vi "PH_ImageOperator.PC Set FF Settings.vi"(0 "i ref in":refnum<vi>, 1 "Calc Fill Factor":bool, 2 "Filter":bool, 3 "Threshold":dbl, 4 "Damage Threshold [J/cm²]":dbl, 5 "error in (no error)":errorcluster) -> (14 "i ref out":refnum<vi>, 19 "error out":errorcluster)   [LabVIEW 2014, in "PH_ImageOperator.lvlib"]
doc: "This VI writes the Fill Factor Measurement settings to own attributes and sets the GUI elements."
uses:
  PH_ImageOperator.lvlib
  PH_Common/PH_Common.lvlib
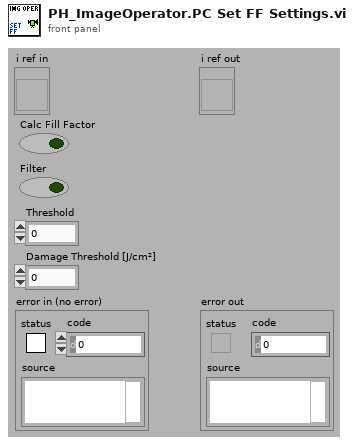
[diagram p1: front panel]
types:
  T1 = typedef "PH_ImageOperator.lvlib/PH_ImageOperator.i attribute.ctl" = cluster{"GUI Refs":cluster{"Delete":refnum<vi>, "Calibration status":refnum<vi>, "BI subtracted":refnum<vi>, "calc Energy":refnum<vi>, "Energy: expected value":refnum<vi>, "Energy: Tolerance":refnum<vi>, "Energy calculated":refnum<vi>, "Energy":refnum<vi>, "calc Beam Anal":refnum<vi>, "Maj Diam 1/esquare":refnum<vi>, "Min Diam 1/esquare":refnum<vi>, "Azi Angle":refnum<vi>, "Min/Maj Diam esquare":refnum<vi>, "Beam analysed":refnum<vi>, "CoG - x":refnum<vi>, "CoG - y":refnum<vi>, "BA: Method":refnum<vi>, "BA: Steps":refnum<vi>, "BA: Factor":refnum<vi>, "calc Traces":refnum<vi>, "Traces: Fit Gauss":refnum<vi>, "Traces calculated":refnum<vi>, "Maj FWHM":refnum<vi>, "Min FWHM":refnum<vi>, "Major Trace":refnum<vi>, "Minor Trace":refnum<vi>, "Maj Fit Order":refnum<vi>, "Min Fit Order":refnum<vi>, "Position calculated":refnum<vi>, "Position":refnum<vi>, "Type":refnum<vi>, "Center":refnum<vi>, "exp - X":refnum<vi>, "exp - Y":refnum<vi>, "Tolerance":refnum<vi>, "f":refnum<vi>, "M":refnum<vi>, "D":refnum<vi>, "q":refnum<vi>, "Dummy Method":refnum<vi>, "Dummy Type":refnum<vi>, "Global On":refnum<vi>, "Traces: No offset":refnum<vi>, "Maj 99%":refnum<vi>, "Min 99%":refnum<vi>, "GUI FF Image":refnum<vi>, "calc Fill Factor":refnum<vi>, "FF calculated":refnum<vi>, "Fill Factor: Filter?":refnum<vi>, "FF: Damage Threshold":refnum<vi>, "FF: Threshold":refnum<vi>, "FF: max allow. Energy":refnum<vi>, "FF: Fillfactor":refnum<vi>, "Calibration data":refnum<vi>}, "List of GUIs":string[], "Calibration":cluster{"Status":T2, "Calibration data":T3, "Calibration Data File":path}, "Final Image":cluster{"BI Subtraction Failure":bool}, "Energy":cluster{"on":bool, "expected value [mJ]":dbl, "Tolerance [%]":dbl, "State":T2, "Energy [mJ]":dbl, "Unit":string, "calculated @":timestamp}, "Beam Analysis":cluster{"on":bool, "Data":T4, "Method":bool, "Steps":i32, "Factor":i32, "ROI":cluster{"Left":i32, "Top":i32, "Right":i32, "Bottom":i32}, "analysed @":timestamp}, "Trace Analysis":cluster{"on":bool, "Fit on":bool, "Maj FWHM":dbl, "Min FWHM":dbl, "Maj Fit Order":i32, "Min Fit Order":i32, "No Offset":bool, "Maj 99%":dbl, "Min 99%":dbl, "Traces":cluster{"XScaleName":string, "Y Scale Minimum":sgl, "Y Scale Maximum":sgl, "X Scale Minimum":sgl, "X Scale Maximum":sgl, "Traces":cluster{"Index":sgl[], "Trace":dbl[]}[]}[], "analysed @":timestamp}, "Position Analysis":cluster{"on":bool, "exp - X":i32, "exp - Y":i32, "focal length [mm]":dbl, "Magnification":dbl, "Delta":dbl, "Theta":dbl, "Tolerance":dbl, "Type":bool, "analysed @":timestamp}, "Fill Factor":cluster{"on":bool, "Filter on?":bool, "Threshold":dbl, "Damage Threshold [J/cm²]":dbl, "Fillfactor":dbl, "Max. allowed Energy [J]":dbl, "calculated @":timestamp}, "Statistician Service ID":i32, "Images":cluster{"Background":T5, "OP":T5, "GUI":T5, "BA: ROI":T5, "Trace: Turn":T5, "FF: Main":T5, "FF: Help":T5, "PSDB: BG":T5, "PSDB: OP":T5, "PSDB: FF":T5}}
  T2 = typedef "PH_StatusHandler.lvlib/PH_StatusHandler.Status.ctl" = i16
  T3 = typedef "PH_ImageCalibrator.lvlib/PH_ImageCalibrator.Calibration Data.ctl" = cluster{"Date":string, "Time":string, "Cam Settings":cluster{"Cam ID":string, "Gain":dbl, "Brightness":dbl, "Shutter":dbl, "Cam Error":bool, "Mode":i32}, "Background Image":cluster{"Image":dbl[][], "Image Error":bool}, "Linear Calibration":cluster{"Calibration Factor":dbl, "not mm or mrad":bool}, "Energy Calibration":cluster{"Calibration Factor":dbl, "no mJ":bool}}
  T4 = typedef "PH_ImageOperator.lvlib/PH_ImageOperator.Beam Analysis Data.ctl" = cluster{"CoG-x":sgl, "CoG-y":sgl, "Maj Dim":dbl, "Min Dim":dbl, "Ellipticity":dbl, "Azimuth Angle [rad]":dbl, "Azi Angle rel to Maj?":bool}
  T5 = typedef "IMAQ Image.ctl" = refnum<image>
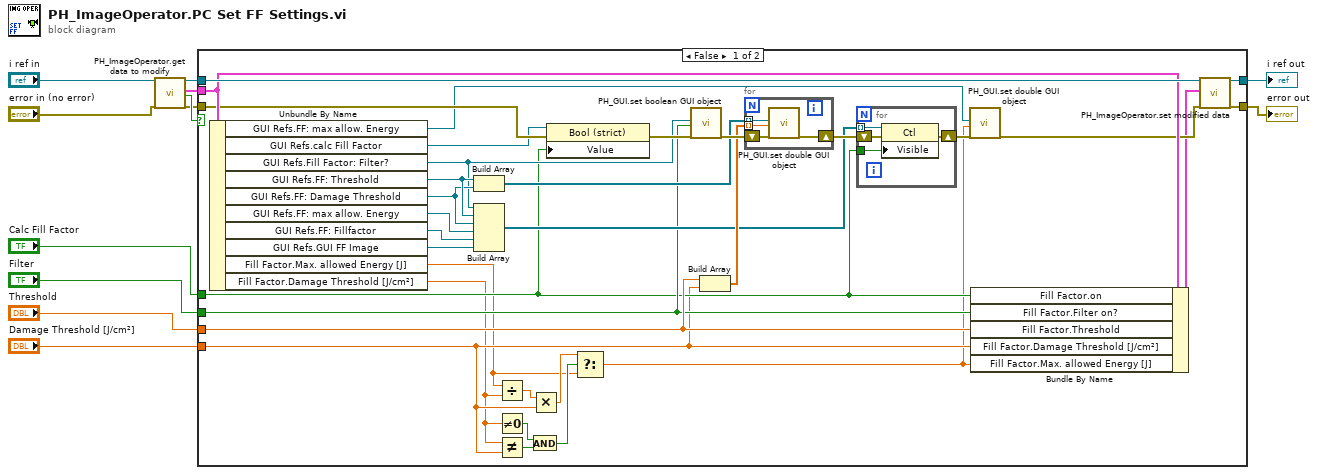
[diagram p0: block diagram]
diagram:
  n1 = call "PH_ImageOperator.get data to modify.vi"("i ref in"="i ref in", "error in (no error)"="error in (no error)") -> ("i ref out"=w4:refnum<vi>, "i attribute"=w9:T1, "timed out"=w8:bool, "error out"=w3:errorcluster)  [unwired: 14 in]
  n2 = case shown="False" w8 {
    tunnel: w3 -> [w32 w55]
    tunnel: w4 -> [w46 w56]
    tunnel: [w45 w56] -> w5
    tunnel: [w44 w55] -> w7
    tunnel: w9 -> [w43 _]
    tunnel: "Calc Fill Factor" -> [w27 _]
    tunnel: "Threshold" -> [w42 _]
    tunnel: "Damage Threshold [J/cm²]" -> [w24 _]
    tunnel: "Filter" -> [w29 _]
    frame False {
      n3 = Unbundle By Name(w43) -> ("GUI Refs.FF: max allow. Energy"=w18:refnum<vi>, "GUI Refs.calc Fill Factor"=w30:refnum<vi>, "GUI Refs.Fill Factor: Filter?"=w28:refnum<vi>, "GUI Refs.FF: Threshold"=w37:refnum<vi>, "GUI Refs.FF: Damage Threshold"=w36:refnum<vi>, "GUI Refs.FF: max allow. Energy"=w35:refnum<vi>, "GUI Refs.FF: Fillfactor"=w34:refnum<vi>, "GUI Refs.GUI FF Image"=w26:refnum<vi>, "Fill Factor.Max. allowed Energy [J]"=w13:dbl, "Fill Factor.Damage Threshold [J/cm²]"=w23:dbl)
      n4 = Build Array(w37, w36) -> (w39:refnum<vi>[])
      n5 = Build Array(w28, w37, w36, w35, w34, w26) -> (w33:refnum<vi>[])
      n6 = Divide(x=w13, y=w23) -> (x/y=w21:dbl)
      n7 = Not Equal To 0?(x=w23) -> (x != 0?=w22:bool)
      n8 = Not Equal?(x=w23, y=w24) -> (x != y?=w25:bool)
      n9 = And(x=w22, y=w25) -> (x .and. y?=w16:bool)
      n10 = Multiply(x=w21, y=w24) -> (x*y=w15:dbl)
      n11 = property class="Bool (strict)"(reference=w30, error in=w32, "Value"=w27) -> (error out=w31:errorcluster)  [unwired: 1 out]
      n12 = Select(t=w15, s=w16, f=w13) -> (s? t:f=w14:dbl)
      n13 = call "PH_GUI.set boolean GUI object.vi"("Boolean Knob GUI Ref"=w28, "Value"=w29, "error in (no error)"=w31) -> ("error out"=w41:errorcluster)  [unwired: 16 in]
      n14 = Build Array(w42, w24) -> (w38:dbl[])
      n15 = for {
        shift-right: [w49] -> w40
        shift-left: w41 -> [w50]
        tunnel: w39 -> [w48] mode=indexing
        tunnel: w38 -> [w47] mode=indexing
        n16 = call "PH_GUI.set double GUI object.vi"("GUI object Ref"=w48, "value"=w47, "error in (no error)"=w50) -> ("error out"=w49:errorcluster)  [unwired: 16 in]
      }
      n17 = for {
        tunnel: w27 -> [w53]
        tunnel: w33 -> [w51] mode=indexing
        shift-right: [w52] -> w20
        shift-left: w40 -> [w54]
        n18 = property class="Ctl"(reference=w51, error in=w54, "Visible"=w53) -> (error out=w52:errorcluster)  [unwired: 1 out]
      }
      n19 = call "PH_GUI.set double GUI object.vi"("GUI object Ref"=w18, "value"=w14, "error in (no error)"=w20) -> ("error out"=w19:errorcluster)  [unwired: 16 in]
      n20 = Bundle By Name(cluster=w43, "Fill Factor.on"=w27, "Fill Factor.Filter on?"=w29, "Fill Factor.Threshold"=w42, "Fill Factor.Damage Threshold [J/cm²]"=w24, "Fill Factor.Max. allowed Energy [J]"=w14) -> (w17:T1)
      n21 = call "PH_ImageOperator.set modified data.vi"("i ref in"=w46, "i attribute"=w17, "error in (no error)"=w19) -> ("i ref out"=w45:refnum<vi>, "error out"=w44:errorcluster)  [unwired: 15 in]
    }
    frame True {
    }
  }
  "error out" <- w7
  "i ref out" <- w5
